vi "string_subset_activity_24.vi"() -> ()   [LabVIEW 2025]
panel:
  in  "Input String":string="VOLTS DC +1.345E+02"
  out "String Subset":string
  out "Number":dbl
  in  "Number Offset":dbl=9.0
  in  "Subset Length":dbl=2.0
  in  "Subset Offset":dbl=6.0
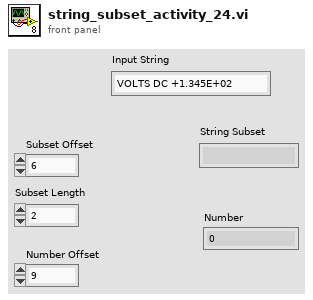
[diagram p1: front panel]
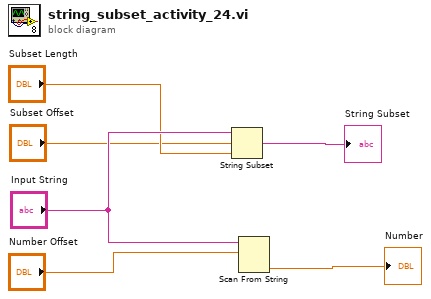
[diagram p0: block diagram]
diagram:
  n1 = String Subset(string="Input String", offset (0)="Subset Offset", length (rest)="Subset Length") -> (substring=→"String Subset":string)
  n2 = Scan From String(input string="Input String", initial scan location="Number Offset") -> (output 1=→"Number":dbl)  [unwired: 3 in, 3 out]
